vi "Cross Power PtByPt.vi"(2 "initialize":bool, 3 "sample length":i32=100, 4 "y":dbl format="%0.2f", 5 "x":dbl format="%0.2f") -> (0 "error":i32, 1 "Sxy":cdb[](array[numeric]))   [LabVIEW 2017, in "NI_PtbyPt.lvlib"]
doc: "Computes the cross power spectrum, <B>Sxy</B>, of the set of input data points specified by <B>sample length</B>."
uses:
  <vilib>/ptbypt/NI_PtbyPt.lvlib
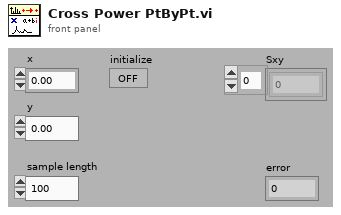
[diagram p1: front panel]
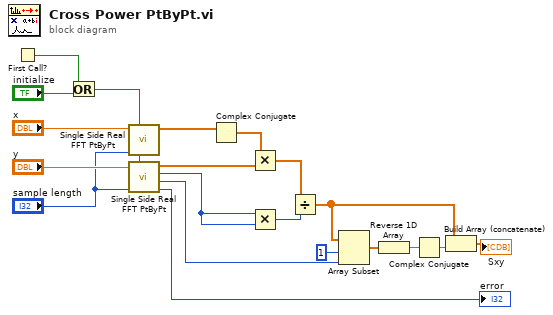
[diagram p0: block diagram]
diagram:
  n1 = First Call?() -> (First Call?: T/F=w1:bool)
  n2 = Or(x=w1, y="initialize") -> (x .or. y?=w2:bool)
  n3 = call <vilib>:"Single Side Real FFT PtByPt.vi"("initialize"=w2, "sample length"="sample length", "input data"="x") -> ("FFT Single Side"=w10:cdb[])  [unwired: 2 in, 3 out]
  n4 = call <vilib>:"Single Side Real FFT PtByPt.vi"("initialize"=w2, "sample length"="sample length", "input data"="y") -> ("error"=→"error":i32, "half length"=w6:i32, "sample length"=w5:i32, "FFT Single Side"=w9:cdb[])  [unwired: 2 in]
  n5 = Complex Conjugate(1:w10) -> (0:w20:cdb[])
  n6 = Multiply(x=w20, y=w9) -> (x*y=w19:cdb[])
  n7 = Multiply(x=w5, y=w5) -> (x*y=w18:i32)
  n8 = Divide(x=w19, y=w18) -> (x/y=w12:cdb[])
  n9 = Array Subset(array=w12, index=1 ("Array Index"), length=w6) -> (w15:cdb[])
  n10 = Reverse 1D Array(array=w15) -> (reversed array=w14:cdb[])
  n11 = Complex Conjugate(1:w14) -> (0:w3:cdb[])
  n12 = Build Array (concatenate)(w12, w3) -> (→"Sxy":cdb[])
